vi "Error.vi"(1 "error in":errorcluster, 2 "code":i32) -> (0 "error out":errorcluster)   [LabVIEW 2010]
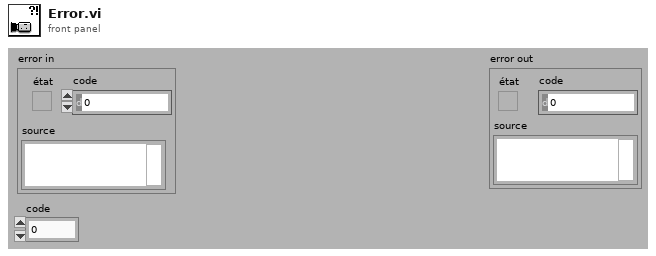
[diagram p1: front panel]
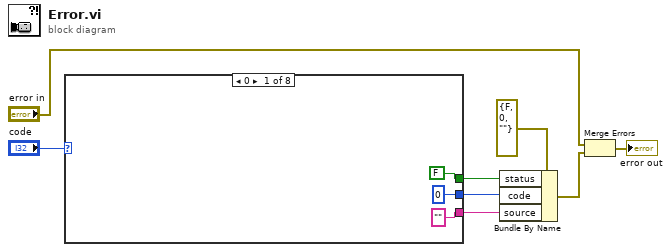
[diagram p0: block diagram]
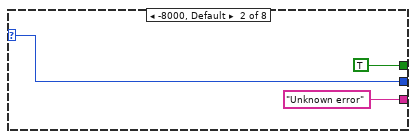
[diagram p2: hidden frame]
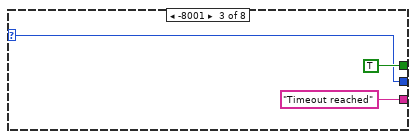
[diagram p3: hidden frame]
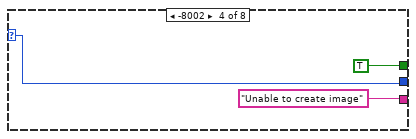
[diagram p4: hidden frame]
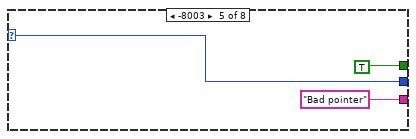
[diagram p5: hidden frame]
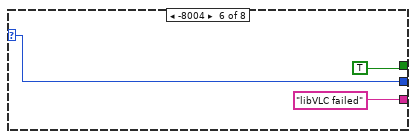
[diagram p6: hidden frame]
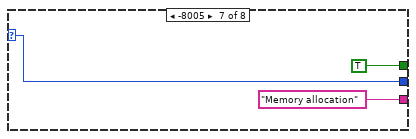
[diagram p7: hidden frame]
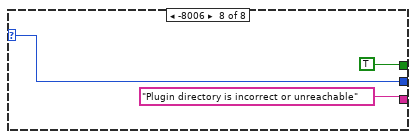
[diagram p8: hidden frame]
diagram:
  n1 = case shown="0" "code" {
    selector: "code" -> [_ w12 w15 w20 w21 w24 w27 w31]
    tunnel: [FALSE ("status") TRUE ("status") TRUE ("status") TRUE ("status") TRUE ("status") TRUE ("status") TRUE ("status") TRUE ("status")] -> w4
    tunnel: [0 ("code") w12 w15 w20 w21 w24 w27 w31] -> w3
    tunnel: ["" ("source") "Unknown error" ("source") "Timeout reached" ("source") "Unable to create image" ("source") "Bad pointer" ("source") "libVLC failed" ("source") "Memory allocation" ("source") "Plugin directory is incorrect or unreachable" ("source")] -> w2
    frame 0 {
    }
    frame -8000, Default {
    }
    frame -8001 {
    }
    frame -8002 {
    }
    frame -8003 {
    }
    frame -8004 {
    }
    frame -8005 {
    }
    frame -8006 {
    }
  }
  n2 = Bundle By Name(cluster=errorcluster {"status"=FALSE, "code"=0, "source"=""} ("error in"), "status"=w4, "code"=w3, "source"=w2) -> (w5:errorcluster)
  n3 = Merge Errors("error in", w5) -> (→"error out":errorcluster)
